vi "URG-04LX-UG01 Initialize.vi"(9 "Acquisition Parameters":T1={"Starting Step"=0, "Ending Step"=768, "Cluster Count"=0, "Scan Interval"=0, "Number of Scans"=0, "Measurement Type"=enum."MS"}, 11 "URG-04LX-UG01 Resource Reference":refnum<visa-resource-name>) -> (0 "error out":errorcluster, 1 "Acquisition Parameters":T1={"Starting Step"=0, "Ending Step"=768, "Cluster Count"=0, "Scan Interval"=0, "Number of Scans"=0, "Measurement Type"=enum."MS"}, 3 "VISA Refnum out":refnum<visa-resource-name>)   [LabVIEW 2018]
doc: "Start a control session with a Hokuyo URG-04LX-UG01 device."
uses:
  Type Definitions/Acquisition Parameters.ctl
  Type Definitions/Measurement Type.ctl
  Type Definitions/Hokuyo Command Parameter.ctl
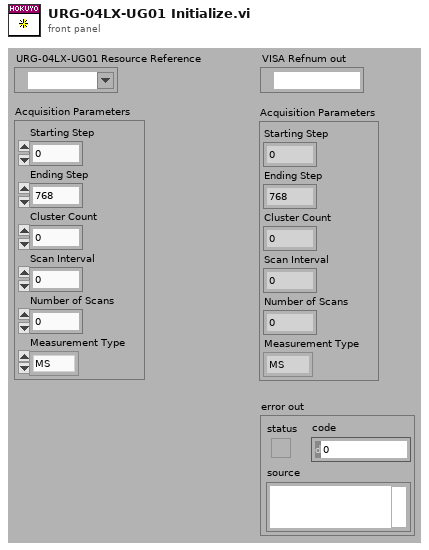
[diagram p1: front panel]
types:
  T1 = typedef "Acquisition Parameters.ctl" = cluster{"Starting Step":i32, "Ending Step":i32, "Cluster Count":i32, "Scan Interval":i32, "Number of Scans":i32, "Measurement Type":T2}
  T2 = typedef "Measurement Type.ctl" = enum16{"MD", "MS"}
  T3 = typedef "Hokuyo Command Parameter.ctl" = cluster{"Device Command":string, "String Characters":string}
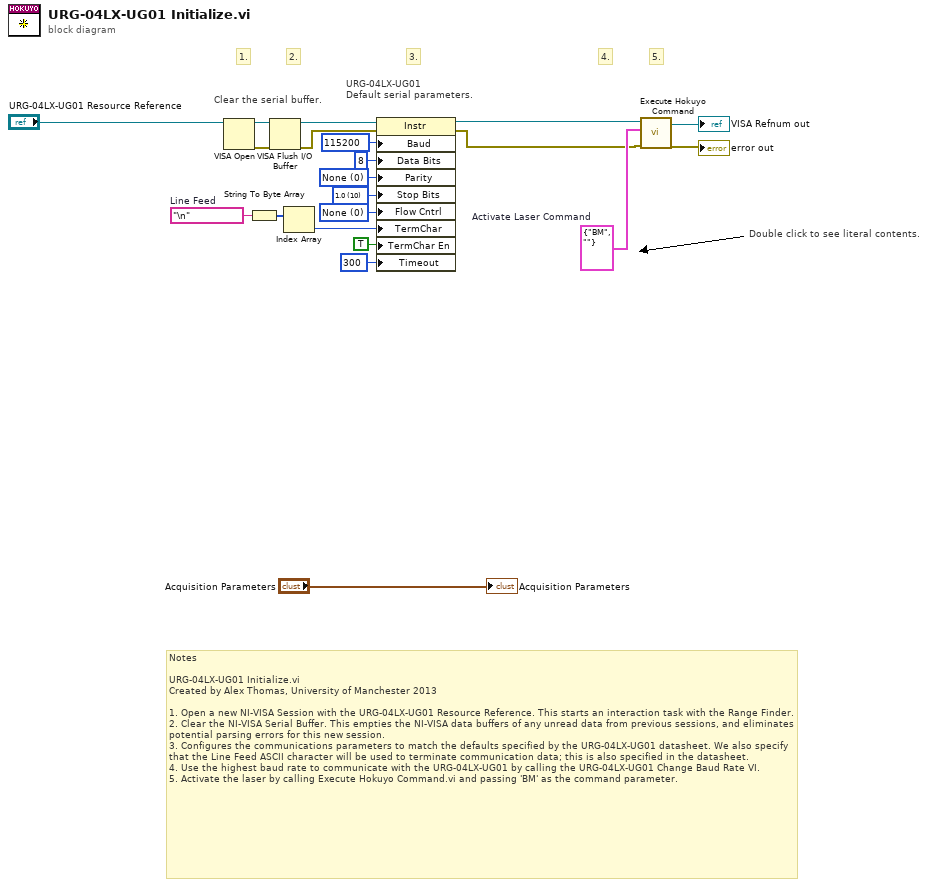
[diagram p0: block diagram]
diagram:
  w18 = T3 {"Device Command"="BM", "String Characters"=""}  # Activate Laser Command
  w9 = "\n"  # Line Feed
  w21 = u16 0 items=["None", "XON/XOFF", "RTS/CTS", "XON/XOFF & RTS/CTS", "DTR/DSR", "XON/XOFF & DTR/DSR"] ("Serial Settings:Flow Control")
  w8 = u16 10 items=["1.0"=10, "1.5"=15, "2.0"=20] ("Serial Settings:Stop Bits")
  w7 = u16 0 items=["None", "Odd", "Even", "Mark", "Space"] ("Serial Settings:Parity")
  # "Double click to see literal contents."
  # "Notes\n\nURG-04LX-UG01 Initialize.vi\nCreated by Alex Thomas, University of Manchester 2013\n\n1. Open a new NI-VISA Session with the URG-04LX-UG01 Resource Reference. This starts an interaction task with the Range Finder.\n2. Clear the NI-VISA Serial Buffer. This empties the NI-VISA data buffers of any unread data from previous sessions, and eliminates potential parsing errors for this new session.\n3. Configures the communications parameters to match the defaults specified by the URG-04LX-UG01 datasheet. We also specify that the Line Feed ASCII character will be used to terminate communication data; this is also specified in the datasheet.\n4. Use the highest baud rate to communicate with the URG-04LX-UG01 by calling the URG-04LX-UG01 Change Baud Rate VI. \n5. Activate the laser by calling Execute Hokuyo Command.vi and passing 'BM' as the command parameter."
  # "5."
  # "4."
  # "3."
  # "2."
  # "1."
  # "Clear the serial buffer."
  # "URG-04LX-UG01\nDefault serial parameters."
  n1 = VISA Open(VISA resource name="URG-04LX-UG01 Resource Reference") -> (VISA resource name=w13:refnum<visa-resource-name>, error out=w14:errorcluster)  [unwired: 4 in]
  n2 = String To Byte Array(string=w9) -> (unsigned byte array=w10:u8[])
  n3 = VISA Flush I/O Buffer(VISA resource name=w13, error in (no error)=w14) -> (VISA resource name out=w16:refnum<visa-resource-name>, error out=w15:errorcluster)  [unwired: 1 in]
  n4 = Index Array(array=w10) -> (element=w11:u8)  [unwired: 1 in]
  n5 = property class="Instr"(reference=w16, error in=w15, "Baud"=u32 115200 ("Serial Settings:Baud Rate"), "Data Bits"=u16 8 ("Serial Settings:Data Bits"), "Parity"=w7, "Stop Bits"=w8, "Flow Cntrl"=w21, "TermChar"=w11, "TermChar En"=TRUE ("Message Based Settings:Termination Character Enable"), "Timeout"=u32 300 ("General Settings:Timeout Value")) -> (reference out=w3:refnum<visa-resource-name>, error out=w2:errorcluster)
  n6 = call "Execute Hokuyo Command.vi"("error in (no error)"=w2, "Hokuyo Command Parameter"=w18, "VISA Refnum in"=w3) -> ("error out"=→"error out":errorcluster, "VISA Refnum out"=→"VISA Refnum out":refnum<visa-resource-name>)  [unwired: 6 in, 1 out]
  "Acquisition Parameters" <- "Acquisition Parameters"
